vi "Arduino Stepper Motor.vi"() -> ()   [LabVIEW 2016, in "LabVIEW Interface for Arduino.lvlib"]
doc: "This example shows how to use the Arduino Stepper Motor API. The fritzing diagram shows use with the EasyStepper 4.3 or 4.4 motor controller."
uses:
  <vilib>/LabVIEW Interface for Arduino/LabVIEW Interface for Arduino.lvlib
panel:
  in  "Stop":bool
  in  "Stepper #":u8=1
  in  "OK Button":bool
  in  "Set Acceleration (0 to disable)":i16
  in  "# of Steps to Move":i16
  in  "Set Speed (Steps per Second)":i16=100
  out "Steps Remaining?":bool
  in  "Dial":i16(knob) scale=0.0..200.0
  in  "error in":errorcluster
  # "Preset Movement"
  # "Interactive Movement"
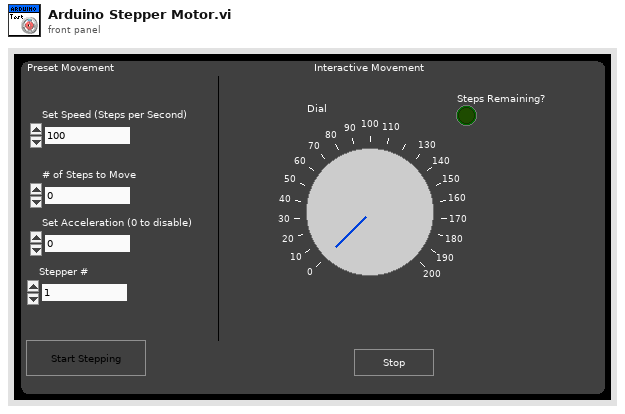
[diagram p1: front panel]
types:
  T1 = typedef "LabVIEW Interface for Arduino.lvlib/Arduino Resource.ctl" = cluster{"VISA resource":refnum<visa-resource-name>, "Board Type":T2, "Connection Type":enum8{"USB / Serial"}, "Bytes Per Packet (15)":u8}
  T2 = typedef "LabVIEW Interface for Arduino.lvlib/Board Type.ctl" = enum16{"Uno", "Dimuelanove w/Atmega 328", "Mega 2560"}
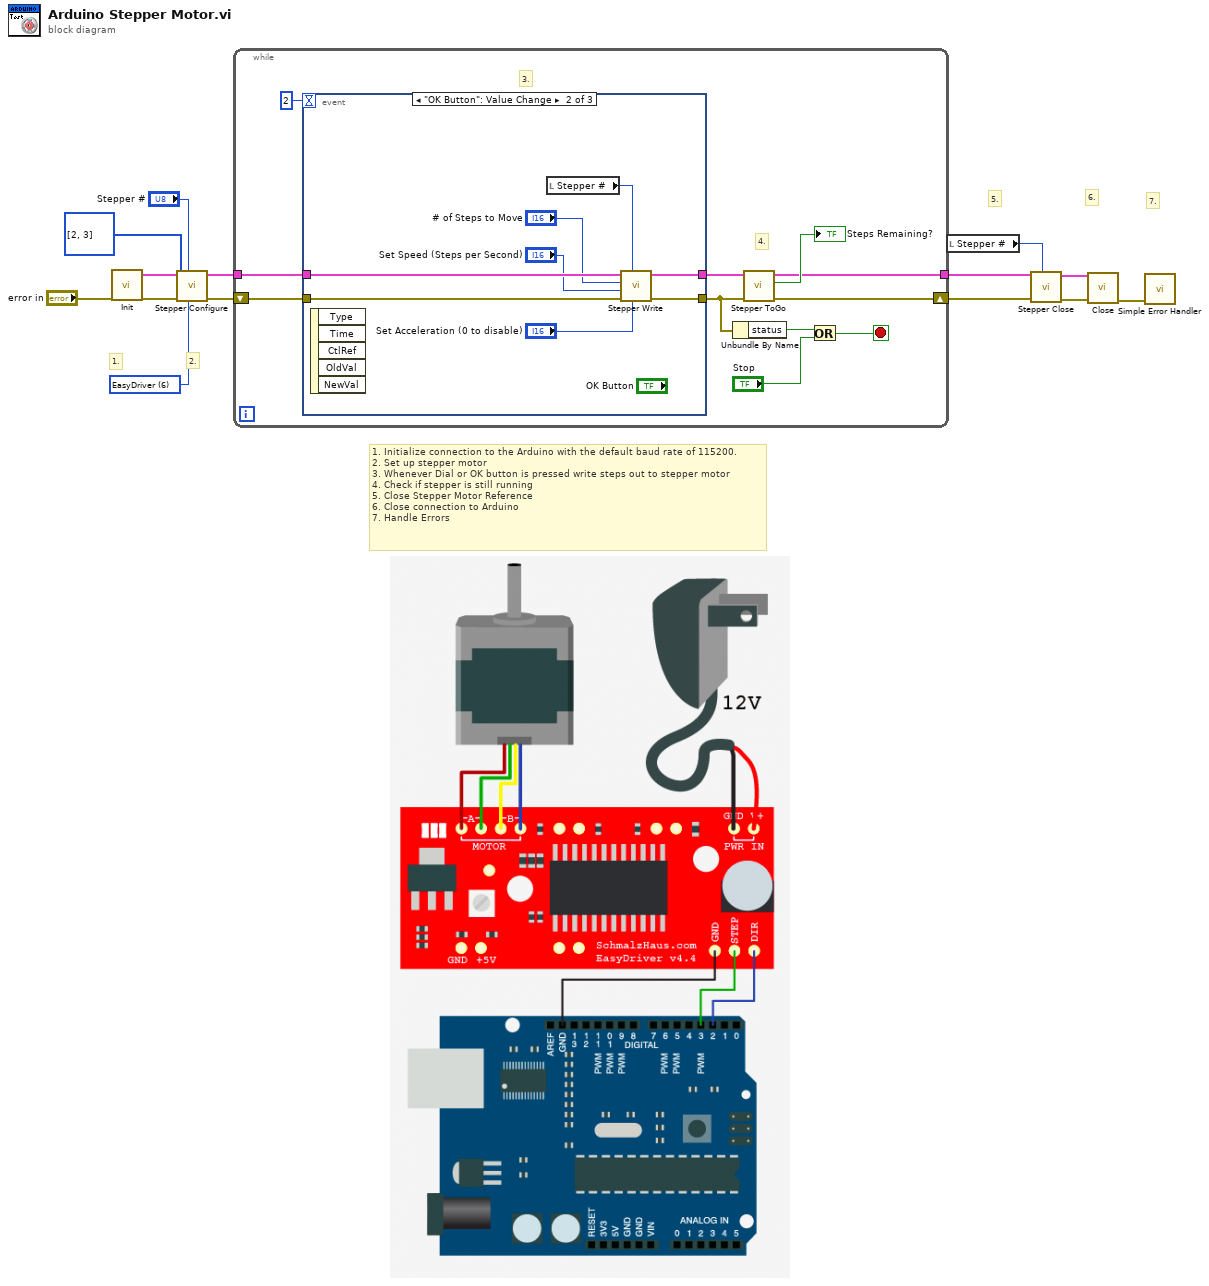
[diagram p0: block diagram]
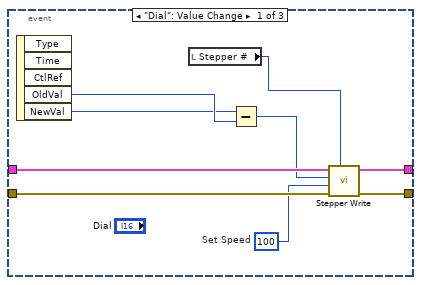
[diagram p2: hidden frame]
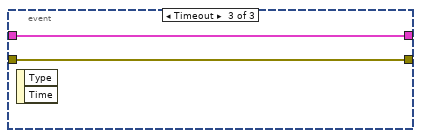
[diagram p3: hidden frame]
diagram:
  w1 = u8 6 items=["2 Wire (Pulse & Direction)"=1, "2 Wire"=2, "4 Wire"=4, "EasyDriver"=6, "AF Motor Shield (Stepper 1 & 2 Only)"=5] ("Control Method")
  # "7."
  # "6."
  # "5."
  # "2."
  # "1."
  # "1. Initialize connection to the Arduino with the default baud rate of 115200.\n2. Set up stepper motor\n3. Whenever Dial or OK button is pressed write steps out to stepper motor\n4. Check if stepper is still running\n5. Close Stepper Motor Reference \n6. Close connection to Arduino\n7. Handle Errors"
  n1 = call <vilib>:"Init.vi"("error in"="error in") -> ("Arduino Resource"=w4:T1, "error out"=w3:errorcluster)  [unwired: 17 in]
  n2 = call <vilib>:"Stepper Configure.vi"("Control Method"=w1, "Stepper #"="Stepper #", "error in"=w3, "Stepper Pins"=u8[] [2, 3], "Arduino Resource"=w4) -> ("error out"=w12:errorcluster, "Arduino Resource Out"=w13:T1)  [unwired: 5 in]
  n3 = while {
    tunnel: w13 -> [w24]
    tunnel: [w18] -> w11
    shift-right: [w16] -> w10
    shift-left: w12 -> [w25]
    stop <- w22 stop-if-true
    # "4."
    # "3."
    n4 = event shown="[1] \"OK Button\": Value Change" {
      selector: _ -> [_ _ _]
      dyn-events: _ -> [_ _ _]
      timeout: 2 -> [_ _ _]
      tunnel: w25 -> [w34 w41 w43]
      tunnel: w24 -> [w33 w39 w44]
      tunnel: [w32 w40 w44] -> w20
      tunnel: [w31 w42 w43] -> w17
      event "Dial": Value Change {
        w28 = i16 100  # Set Speed
        n5 = event-data() -> ("OldVal"=w30:i16, "NewVal"=w29:i16)  [unwired: 1 in, 3 out]
        n6 = local read "Stepper #"() -> (w26:u8)
        n7 = Subtract(x=w29, y=w30) -> (x-y=w27:i16)
        n8 = call <vilib>:"Stepper Write.vi"("Stepper #"=w26, "error in"=w34, "Set Speed (Steps per Second)"=w28, "# of Steps to Move"=w27, "Arduino Resource"=w33) -> ("error out"=w31:errorcluster, "Arduino Resource Out"=w32:T1)  [unwired: 5 in]
      }
      event "OK Button": Value Change {
        n9 = event-data() -> ()  [unwired: 1 in, 5 out]
        n10 = local read "Stepper #"() -> (w35:u8)
        n11 = call <vilib>:"Stepper Write.vi"("Set Acceleration (0 to disable)"="Set Acceleration (0 to disable)", "Stepper #"=w35, "error in"=w41, "Set Speed (Steps per Second)"="Set Speed (Steps per Second)", "# of Steps to Move"="# of Steps to Move", "Arduino Resource"=w39) -> ("error out"=w42:errorcluster, "Arduino Resource Out"=w40:T1)  [unwired: 4 in]
      }
      event Timeout {
        n12 = event-data() -> ()  [unwired: 1 in, 2 out]
      }
    }
    n13 = Unbundle By Name(w17) -> ("status"=w21:bool)
    n14 = call <vilib>:"Stepper ToGo.vi"("error in"=w17, "Arduino Resource"=w20) -> ("error out"=w16:errorcluster, "Steps Remaining?"=→"Steps Remaining?":bool, "Arduino Resource Out"=w18:T1)  [unwired: 6 in, 1 out]
    n15 = Or(x=w21, y="Stop") -> (x .or. y?=w22:bool)
  }
  n16 = local read "Stepper #"() -> (w5:u8)
  n17 = call <vilib>:"Stepper Close.vi"("Stepper #"=w5, "error in"=w10, "Arduino Resource"=w11) -> ("error out"=w9:errorcluster, "Arduino Resource Out"=w8:T1)  [unwired: 7 in]
  n18 = call <vilib>:"Close.vi"("Arduino Resource"=w8, "error in"=w9) -> ("error out"=w14:errorcluster)  [unwired: 13 in]
  n19 = call <vilib>:"Simple Error Handler.vi"("error in (no error)"=w14) -> ()  [unwired: 4 in, 5 out]
